vi "simulacion.vi"() -> ()   [LabVIEW 2020]
panel:
  in  "stop":bool
  out "Waveform Chart":dynamicdata(graph)
  out "TEst":string[][](array[string])
  out "text":string
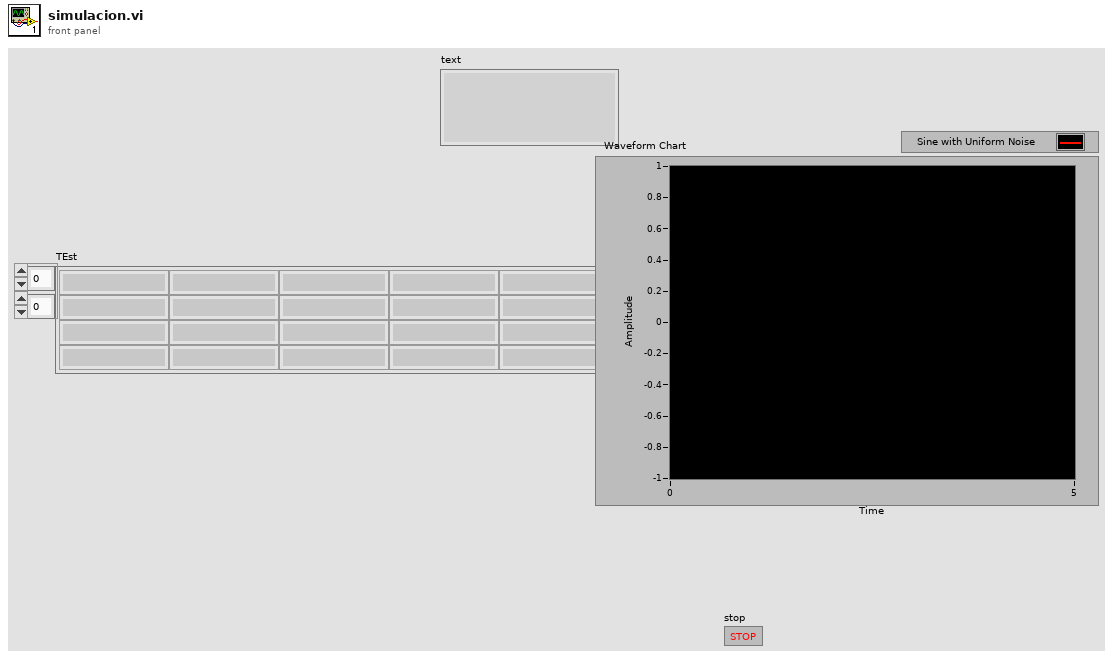
[diagram p1: front panel]
types:
  T1 = enum16{"open", "replace", "create", "open or create", "replace or create", "replace or create with confirmation"}
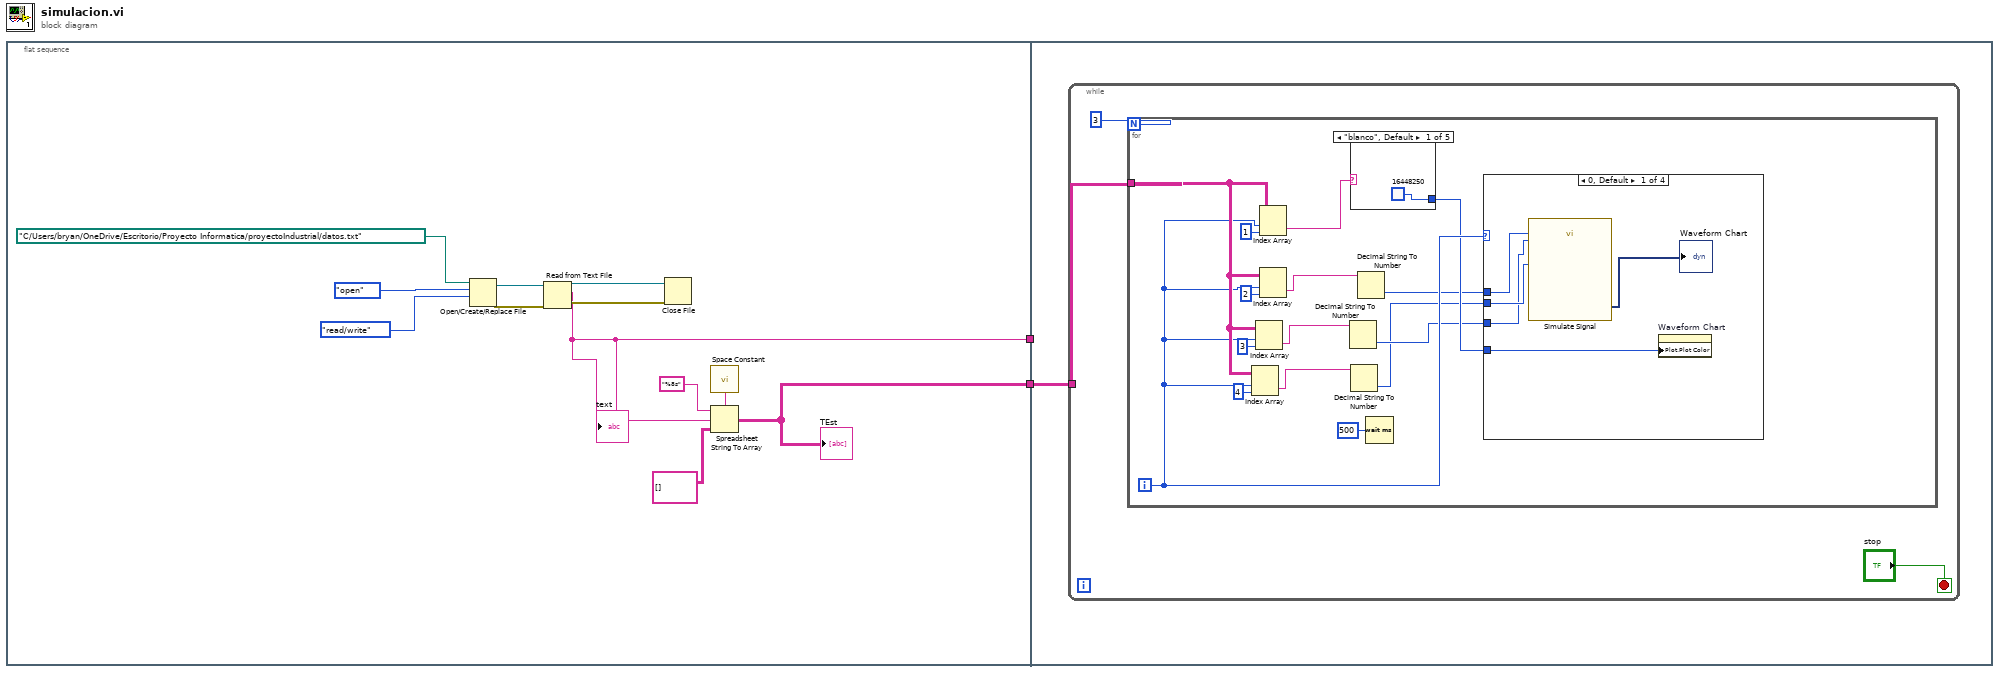
[diagram p0: block diagram]
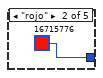
[diagram p2: hidden frame]
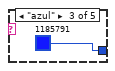
[diagram p3: hidden frame]
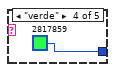
[diagram p4: hidden frame]
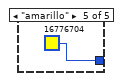
[diagram p5: hidden frame]
diagram:
  n1 = flat-sequence {
    tunnel: [w7] -> w2
    tunnel: [w3] -> w1
    tunnel: w2 -> [_]
    tunnel: w1 -> [w15]
    frame #0 {
      n2 = Open/Create/Replace File(file path (use dialog)=path "C:/Users/bryan/OneDrive/Escritorio/Proyecto Informatica/proyectoIndustrial/datos.txt", operation (0:open)=T1."open", access (0:read/write)=enum16{"read/write", "read-only", "write-only"}."read/write") -> (refnum out=w11:refnum<file>, error out=w10:errorcluster)  [unwired: 3 in, 1 out]
      n3 = Read from Text File(file (use dialog)=w11, error in=w10) -> (refnum out=w9:refnum<file>, text=w7:string, error out=w8:errorcluster)  [unwired: 2 in, 1 out]
      "text" <- w7
      n4 = Close File(refnum=w9, error in=w8) -> ()  [unwired: 2 out]
      n5 = call <vilib>:"Space Constant.vi"() -> ("String"=w4:string)
      n6 = Spreadsheet String To Array(delimiter (Tab)=w4, format string="%8s", spreadsheet string=w7, array type (2D Dbl)=string[][] []) -> (array=w3:string[][])
      "TEst" <- w3
    }
    frame #1 {
      n7 = while {
        tunnel: w15 -> [w17]
        stop <- "stop" stop-if-true
        n8 = for {
          N: 3 -> [_]
          tunnel: w17 -> [w33]
          i -> [w31]
          n9 = Index Array(array=w33, index (row)=w31, index (col)=4 ("disabled index (col)")) -> (element=w21:string)
          n10 = Index Array(array=w33, index (row)=w31, index (col)=3 ("disabled index (col)")) -> (element=w23:string)
          n11 = Index Array(array=w33, index (row)=w31, index (col)=1 ("disabled index (col)")) -> (element=w27:string)
          n12 = Index Array(array=w33, index (row)=w31, index (col)=2 ("disabled index (col)")) -> (element=w25:string)
          n13 = Decimal String To Number(string=w23) -> (number=w22:i32)  [unwired: 2 in, 1 out]
          n14 = case shown="\"blanco\", Default" w27 {
            tunnel: [u32 16448250 ("Plot.Plot Color") u32 16715776 ("Plot.Plot Color") u32 1185791 ("Plot.Plot Color") u32 2817859 ("Plot.Plot Color") u32 16776704 ("Plot.Plot Color")] -> w26
            frame "blanco", Default {
            }
            frame "rojo" {
            }
            frame "azul" {
            }
            frame "verde" {
            }
            frame "amarillo" {
            }
          }
          n15 = Decimal String To Number(string=w21) -> (number=w20:i32)  [unwired: 2 in, 1 out]
          n16 = Decimal String To Number(string=w25) -> (number=w24:i32)  [unwired: 2 in, 1 out]
          n17 = Wait (ms)(milliseconds to wait=u32 500) -> ()  [unwired: 1 out]
          n18 = case shown="0, Default" w31 {
            tunnel: w26 -> [w43 _ _ _]
            tunnel: w24 -> [w42 _ _ _]
            tunnel: w22 -> [w40 _ _ _]
            tunnel: w20 -> [w41 _ _ _]
            frame 0, Default {
              n19 = call "Simulate Signal"("Frequency"=w42, "Amplitude"=w40, "Noise amplitude"=w41) -> ("Sine with Uniform Noise"=→"Waveform Chart":dynamicdata)  [unwired: 11 in, 1 out]
              n20 = property on="Waveform Chart" class="WFChart (strict)"("Plot.Plot Color"=w43) -> ()  [unwired: 2 in, 2 out]
            }
            frame 3 {
            }
            frame 1 {
            }
            frame 2 {
            }
          }
        }
      }
    }
  }
